vi "set_subcomponents.vi"(8 "error in (no error)":errorcluster, 10 "subcomponents":refnum<class "GenericComponent.lvclass">[](array[class]), 11 "ScanHeadDL090202 in":refnum<class "ScanHeadDL090202.lvclass">) -> (0 "error out":errorcluster, 3 "ScanHeadDL090202 out":refnum<class "ScanHeadDL090202.lvclass">)   [LabVIEW 2010, in "ScanHeadDL090202.lvclass"]
uses:
  ScanHeadDL090202.lvclass
  common/classes/GenericComponent/GenericComponent/GenericComponent.lvclass
  Shutter/GenericShutter/GenericShutter/GenericShutter.lvclass
  Clock/GenericClock/GenericClock/GenericClock.lvclass
  SignalWriter/GenericSignalWriter/GenericSignalWriter/GenericSignalWriter.lvclass
  ScanHeadDL090202.lvclass/ScanHeadDL090202.ctl
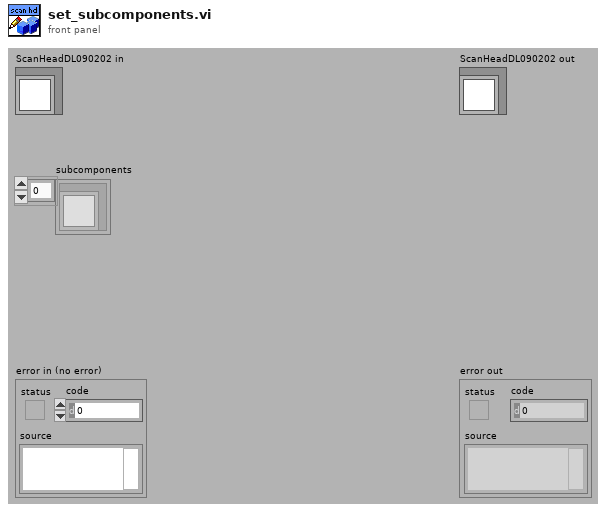
[diagram p1: front panel]
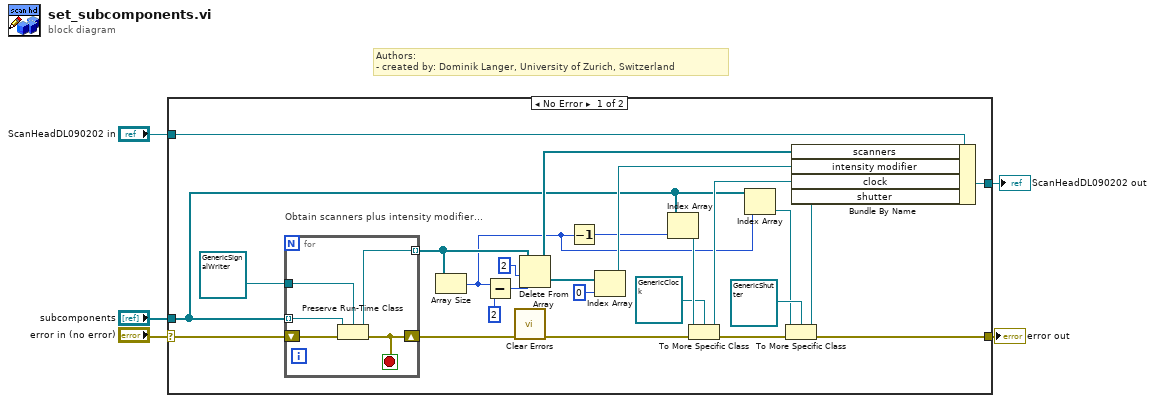
[diagram p0: block diagram]
diagram:
  # "Authors: \n- created by: Dominik Langer, University of Zurich, Switzerland"
  n1 = case shown="No Error" "error in (no error)" {
    selector: "error in (no error)" -> [w30 w37]
    tunnel: "ScanHeadDL090202 in" -> [w29 w36]
    tunnel: "subcomponents" -> [w11 _]
    tunnel: [w12 w37] -> w2
    tunnel: [w24 w36] -> w1
    frame No Error {
      n2 = for "Obtain scanners plus intensity modifier..." {
        shift-right: [w32] -> w25
        shift-left: w30 -> [w35]
        tunnel: w11 -> [w34] mode=indexing
        tunnel: [w33] -> w27 mode=indexing
        tunnel: refnum<class "GenericSignalWriter.lvclass"> refnum ("write signals") -> [w31]
        stop <- w32 stop-if-true
        n3 = Preserve Run-Time Class(object in=w34, error in=w35, 2:w31) -> (object out=w33:refnum<class "GenericSignalWriter.lvclass">, error out=w32:errorcluster)
      }
      n4 = Array Size(array=w27) -> (size(s)=w6:i32)
      n5 = Subtract(x=w6, y=2) -> (x-y=w8:i32)
      n6 = call <vilib>:"Clear Errors.vi"("error in (no error)"=w25) -> ("error out"=w17:errorcluster)  [unwired: 6 in]
      n7 = Delete From Array(array=w27, length=2, index=w8) -> (deleted portion=w21:refnum<class "GenericSignalWriter.lvclass">[], array with subset deleted=w28:refnum<class "GenericSignalWriter.lvclass">[])
      n8 = Decrement(x=w6) -> (x-1=w7:i32)
      n9 = Index Array(array=w21, index=0) -> (element=w20:refnum<class "GenericSignalWriter.lvclass">)
      n10 = Index Array(array=w11, index=w7) -> (element=w19:refnum<class "GenericComponent.lvclass">)
      n11 = To More Specific Class(target class=refnum<class "GenericClock.lvclass"> refnum ("subcomponents.clock"), reference=w19, error in=w17) -> (specific class reference=w16:refnum<class "GenericClock.lvclass">, error out=w13:errorcluster)
      n12 = Index Array(array=w11, index=w6) -> (element=w10:refnum<class "GenericComponent.lvclass">)
      n13 = To More Specific Class(target class=refnum<class "GenericShutter.lvclass"> refnum ("subcomponents.shutter"), reference=w10, error in=w13) -> (specific class reference=w14:refnum<class "GenericShutter.lvclass">, error out=w12:errorcluster)
      n14 = Bundle By Name(cluster=w29, "scanners"=w28, "intensity modifier"=w20, "clock"=w16, "shutter"=w14) -> (w24:refnum<class "ScanHeadDL090202.lvclass">)
    }
    frame Error {
    }
  }
  "error out" <- w2
  "ScanHeadDL090202 out" <- w1
